vi "write memory.vi"(8 "error in (no error)":errorcluster, 10 "IQ data":u64[](array[numeric]), 11 "p2p vst in":refnum<class "p2p vst.lvclass">) -> (0 "error out":errorcluster, 3 "p2p vst out":refnum<class "p2p vst.lvclass">)   [LabVIEW 2021, in "p2p vst.lvclass"]
uses:
  p2p vst.lvclass
  p2p vst.lvclass/p2p vst.ctl
  <vilib>/rvi/interface/common/niFpgaWaitOnOcc.vi
  <vilib>/Utility/error.llb/Error Cluster From Error Code.vi
  <vilib>/rvi/errors/niLvFpgaAdjustHostInterfaceError.vi
  <vilib>/rvi/interface/nirviMethod/nirviMethod.xnode
  <vilib>/rvi/errors/niLvFpgaMergeErrorWithErrorCode.vi
  <vilib>/FPGAPlugInAG/Dynamic/niLvFpga_ConfigureFifo_Dynamic.vi
  <vilib>/FPGAPlugInAG/Dynamic/niLvFpga_WriteFifo_Dynamic.vi
  <vilib>/FPGAPlugInAG/Dynamic/niLvFpga_StopFifo_Dynamic.vi
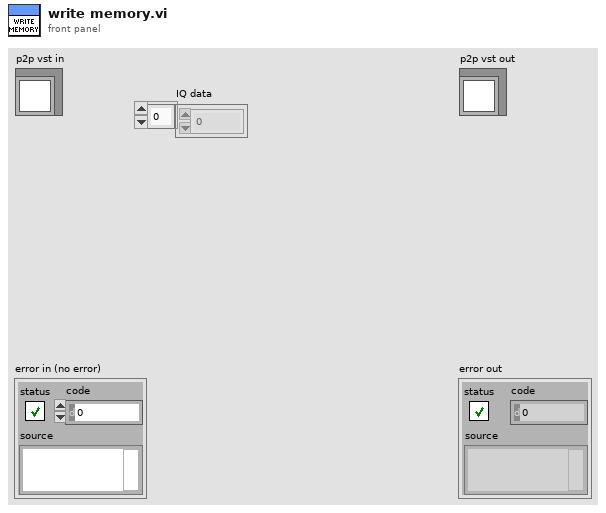
[diagram p1: front panel]
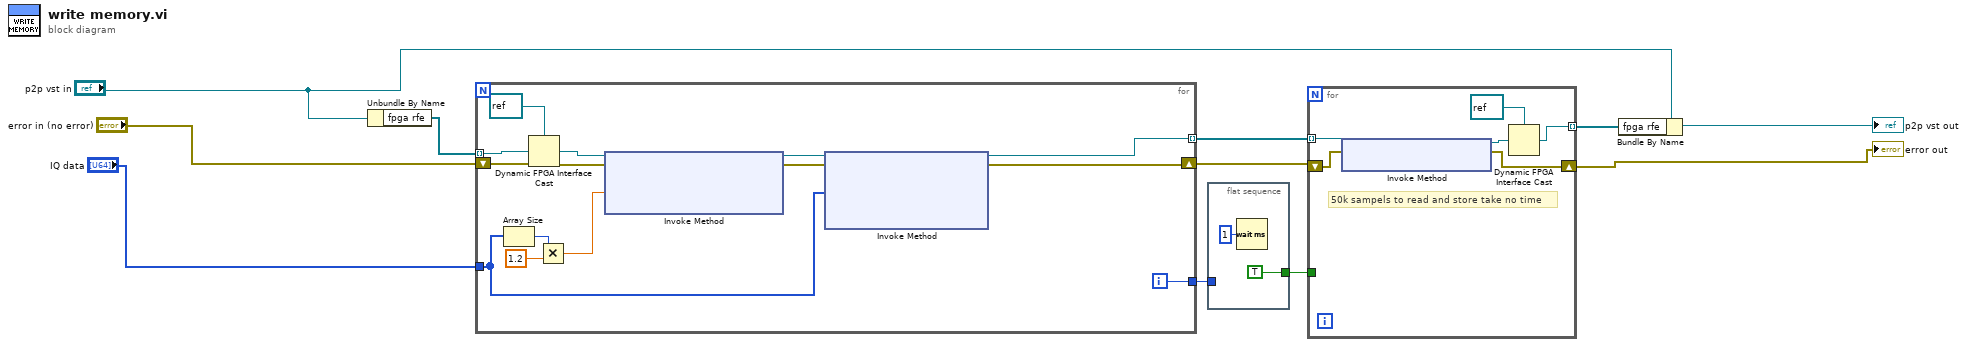
[diagram p0: block diagram]
diagram:
  n1 = Unbundle By Name("p2p vst in") -> ("fpga rfe"=w11:refnum<k20>[])
  n2 = for {
    tunnel: w11 -> [w14] mode=indexing
    shift-right: [w23] -> w8
    shift-left: "error in (no error)" -> [w19]
    tunnel: [w24] -> w10 mode=indexing
    tunnel: [w16] -> w6
    tunnel: "IQ data" -> [w15]
    i -> [w16]
    n3 = Array Size(array=w15) -> (size(s)=w22:i32)
    n4 = Dynamic FPGA Interface Cast(Session In=refnum<k20> refnum ("Type"), Type=w14) -> (Session Out=w13:refnum<k20>)
    n5 = Multiply(x=w22, y=1.2) -> (x*y=w21:dbl)
    n6 = xnode "Invoke Method"("FPGA VI Reference In"=w13, "error in"=w19, "Requested Depth"=w21) -> ("FPGA VI Reference Out"=w18:refnum<k20>, "error out"=w17:errorcluster)  [unwired: 1 out]
    n7 = xnode "Invoke Method"("FPGA VI Reference In"=w18, "error in"=w17, "Data"=w15) -> ("FPGA VI Reference Out"=w24:refnum<k20>, "error out"=w23:errorcluster)  [unwired: 1 in, 1 out]
  }
  n8 = flat-sequence {
    tunnel: [TRUE] -> w7
    tunnel: w6 -> [_]
    frame #0 {
      n9 = Wait (ms)(milliseconds to wait=u32 1) -> ()  [unwired: 1 out]
    }
  }
  n10 = for {
    tunnel: w10 -> [w32] mode=indexing
    tunnel: [w28] -> w9 mode=indexing
    shift-right: [w30] -> w5
    shift-left: w8 -> [w31]
    tunnel: w7 -> [_]
    # "50k sampels to read and store take no time"
    n11 = xnode "Invoke Method"("FPGA VI Reference In"=w32, "error in"=w31) -> ("FPGA VI Reference Out"=w29:refnum<k20>, "error out"=w30:errorcluster)
    n12 = Dynamic FPGA Interface Cast(Session In=refnum<k20> refnum ("FPGA VI Reference Out"), Type=w29) -> (Session Out=w28:refnum<k20>)
  }
  "error out" <- w5
  n13 = Bundle By Name(cluster="p2p vst in", "fpga rfe"=w9) -> (→"p2p vst out":refnum<class "p2p vst.lvclass">)
